vi "Write chirp duration [s].vi"(8 "error in (no error)":errorcluster, 11 "ChirpEIS in":refnum<class "ChirpEIS.lvclass">) -> (0 "error out":errorcluster, 2 "Less than Max":bool, 3 "ChirpEIS out":refnum<class "ChirpEIS.lvclass">)   [LabVIEW 2014, in "ChirpEIS.lvclass"]
uses:
  ChirpEIS.lvclass
  ChirpEIS.lvclass/ChirpEIS.ctl
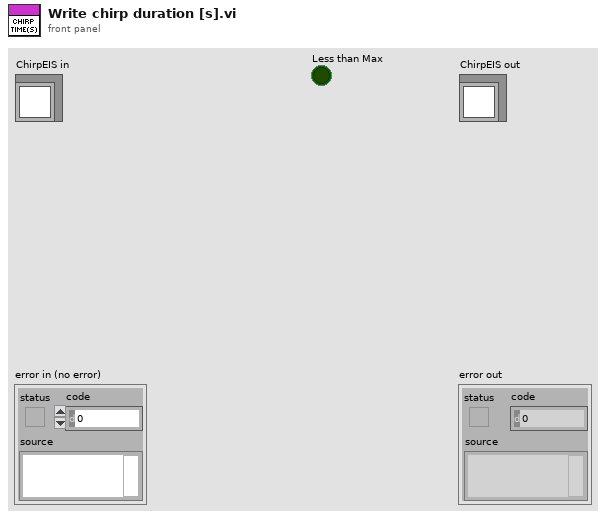
[diagram p1: front panel]
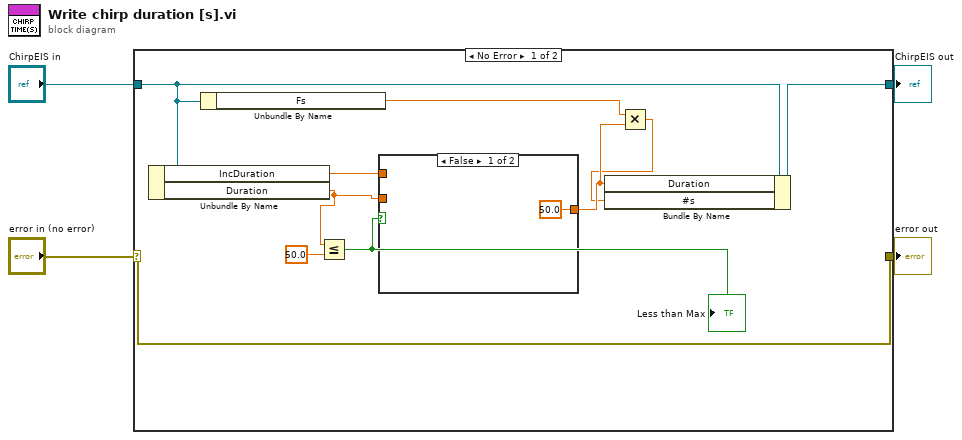
[diagram p0: block diagram]
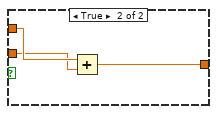
[diagram p2: hidden frame]
diagram:
  n1 = case shown="No Error" "error in (no error)" {
    selector: "error in (no error)" -> [w14 w19]
    tunnel: [w14 w19] -> w3
    tunnel: [w13 w20] -> w1
    tunnel: "ChirpEIS in" -> [w8 w20]
    frame No Error {
      n2 = Unbundle By Name(w8) -> ("IncDuration"=w10:dbl, "Duration"=w9:dbl)
      n3 = Unbundle By Name(w8) -> ("Fs"=w7:dbl)
      n4 = Less Or Equal?(x=w9, y=50.0) -> (x <= y?=w11:bool)
      "Less than Max" <- w11
      n5 = case shown="False" w11 {
        tunnel: w10 -> [_ w18]
        tunnel: w9 -> [_ w17]
        tunnel: [50.0 w16] -> w6
        frame False {
        }
        frame True {
          n6 = Add(x=w18, y=w17) -> (x+y=w16:dbl)
        }
      }
      n7 = Multiply(x=w7, y=w6) -> (x*y=w5:dbl)
      n8 = Bundle By Name(cluster=w8, "Duration"=w6, "#s"=w5) -> (w13:refnum<class "ChirpEIS.lvclass">)
    }
    frame Error {
    }
  }
  "error out" <- w3
  "ChirpEIS out" <- w1
